vi "Teleop.vi"(10 "Match Info":T2={"Autonomous Elapsed Seconds"=0.0, "TeleOp Elapsed Seconds"=0.0, "Disabled Elapsed Seconds"=0.0, "Visited Autonomous"=FALSE, "Visited TeleOp"=FALSE, "Visited Disabled"=FALSE, "Autonomous Settings"={"Autonomous Style"=enum."Independent", "VI Refnum"=refnum}}, 11 "Call Context":T3) -> ()   [LabVIEW 2011]
doc: "This VI is called for each TeleOp packet received from the DS where the robot is not disabled. It is often used to read from the joysticks and update I/O or to update setpoints for timed control loops. It should complete and return within 20 milliseconds or it may miss DS packets."
uses:
  <vilib>/Rock Robotics/WPI/DriverStation/WPI_DriverStationDerivedRobotMode.ctl
  <vilib>/Rock Robotics/WPI/DriverStation/WPI_DriverStationMatch Info.ctl
  <vilib>/Rock Robotics/WPI/Relay/WPI_RelayValue.ctl
  Robot Global Data.vi
  <vilib>/ptbypt/NI_PtbyPt.lvlib
panel:
  in  "AutoSearch?":bool
  in  "MotorPower":dbl
  in  "Slide":dbl(slide) scale=400.0..2000.0
  out "Numeric":dbl
  out "Knob":dbl(knob) scale=0.0..360.0
  in  "RelayValue":T1
  out "Value 5":bool
  out "Value 4":bool
  out "Value 3":bool
  out "Value 2":bool
  out "Value":bool
  in  "top":bool=TRUE
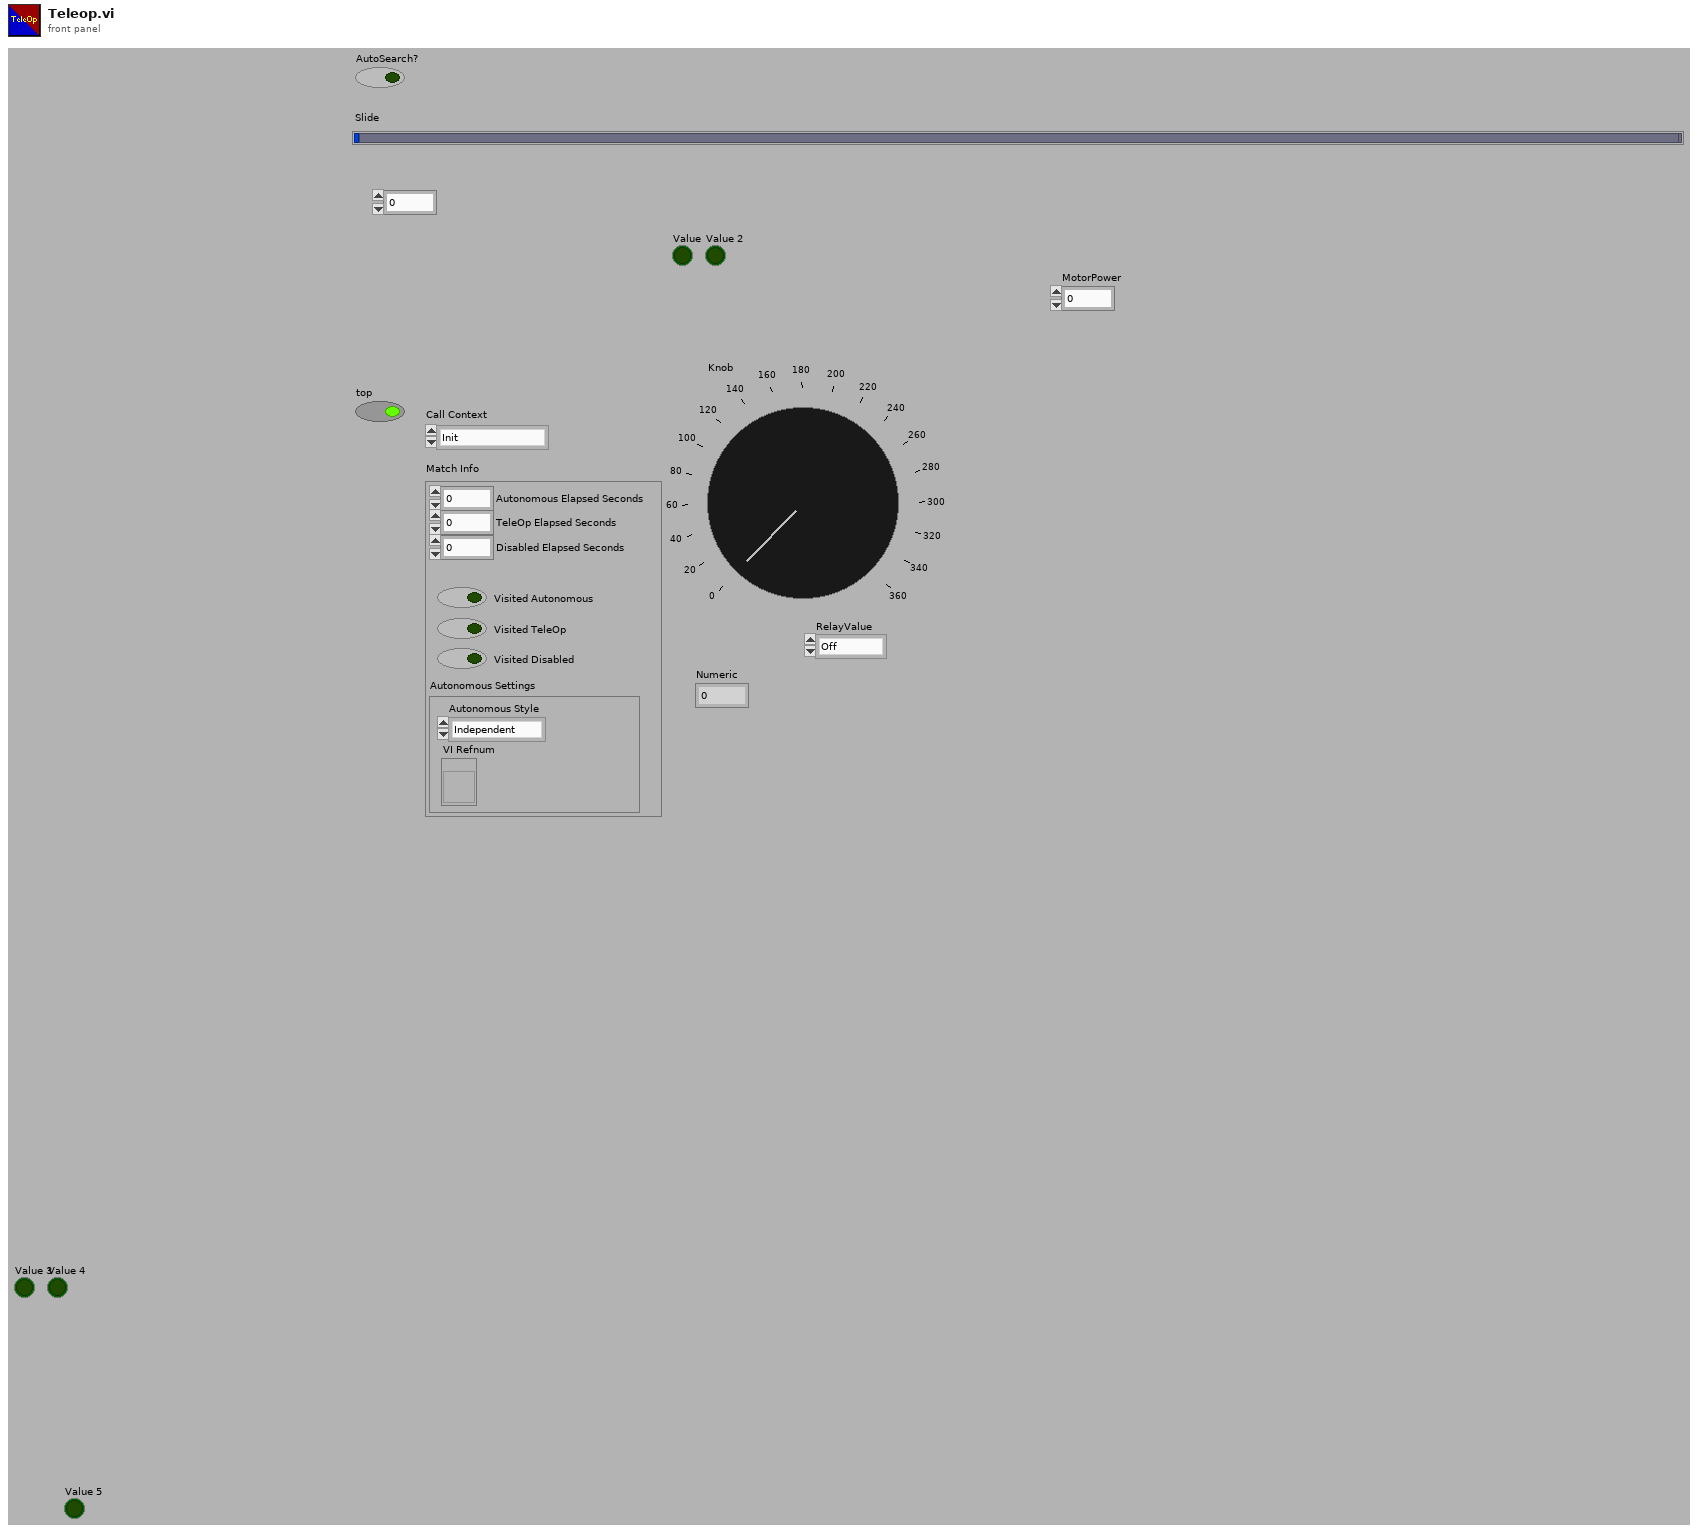
[diagram p1: front panel]
types:
  T1 = typedef "WPI_RelayValue.ctl" = enum16{"Off", "On", "Forward", "Reverse"}
  T2 = typedef "WPI_DriverStationMatch Info.ctl" = cluster{"Autonomous Elapsed Seconds":dbl, "TeleOp Elapsed Seconds":dbl, "Disabled Elapsed Seconds":dbl, "Visited Autonomous":bool, "Visited TeleOp":bool, "Visited Disabled":bool, "Autonomous Settings":cluster{"Autonomous Style":enum16{"Iterative", "Independent"}, "VI Refnum":refnum<vi>}}
  T3 = typedef "WPI_DriverStationDerivedRobotMode.ctl" = enum16{"Init", "Execute", "Stop"}
  T4 = typedef "WPI_RelayDevRef.ctl" = cluster{"DevStatus":errorcluster, "Relay Channel":T5, "Digital Module":T6, "Relay Direction":T7}
  T5 = typedef "FPGA_DIORelayChannel.ctl" = enum8{"Relay 1", "Relay 2", "Relay 3", "Relay 4", "Relay 5", "Relay 6", "Relay 7", "Relay 8", "Invalid"}
  T6 = typedef "FPGA_TypedefDigitalModule.ctl" = enum16{"Digital Module 1", "Digital Module 2"}
  T7 = typedef "WPI_RelayDirection.ctl" = enum16{"Both directions", "Forward only", "Reverse only"}
  T8 = typedef "WPI_AnalogChannelDevRef.ctl" = cluster{"DevStatus":errorcluster, "Analog Module":T9, "Analog Channel":T10}
  T9 = typedef "FPGA_TypedefAnalogModule.ctl" = enum16{"Analog Module 1", "Analog Module 2"}
  T10 = typedef "FPGA_AIChannel.ctl" = enum8{"AI 1", "AI 2", "AI 3", "AI 4", "AI 5", "AI 6", "AI 7", "AI 8", "Invalid"}
  T11 = typedef "WPI_DigitalInputDevRef.ctl" = cluster{"DevStatus":errorcluster, "DIO Channel":T12, "Digital Module":T6}
  T12 = typedef "FPGA_DIOChannel.ctl" = enum8{"DIO 1", "DIO 2", "DIO 3", "DIO 4", "DIO 5", "DIO 6", "DIO 7", "DIO 8", "DIO 9", "DIO 10", "DIO 11", "DIO 12", "DIO 13", "DIO 14", "Invalid"}
  T13 = cluster{"Position":cluster{"X":dbl, "Y":dbl}, "Distance (m)":dbl, "Target Found?":bool}
  T14 = typedef "WPI_ServoDeviceRef.ctl" = cluster{"DeviceStatus":errorcluster, "Digital Module":T6, "PWM Channel":T15, "DeadBand":T16}
  T15 = typedef "FPGA_DIOPWMChannel.ctl" = enum8{"PWM 1", "PWM 2", "PWM 3", "PWM 4", "PWM 5", "PWM 6", "PWM 7", "PWM 8", "PWM 9", "PWM 10", "Invalid"}
  T16 = typedef "WPI_PWMDeadband.ctl" = cluster{"Name":string, "maxPositivePwm":i32, "minPositivePwm":i32, "centerPwm":i32, "maxNegativePwm":i32, "minNegativePwm":i32, "angularRange":u16}
  T17 = typedef "WPI_MotorControlDeviceRef.ctl" = cluster{"DeviceStatus":errorcluster, "Type":enum16{"PWM", "CAN"}, "PWM":cluster{"Digital Module":T6, "PWM Channel":T15, "DeadBand":T16}, "CAN":cluster{"Device Number":u8, "Control Mode":T18, "Semaphore":T19, "Max Vout":dbl}, "Invert":bool, "TransformRef":T20, "InvTransformRef":T20}
  T18 = typedef "WPI_CANJaguar_ControlMode.ctl" = enum8{"Percent VBus", "Current", "Speed", "Position", "Voltage"}
  T19 = typedef "Semaphore RefNum" = refnum<k1>
  T20 = typedef "WPI_PWMTransform_ConPane.ctl" = refnum<vi>
  T21 = typedef "WPI_JoystickDevRef.ctl" = cluster{"Device":T22}
  T22 = typedef "WPI_JoystickDeviceEnum.ctl" = enum16{"USB 1", "USB 2", "USB 3", "USB 4", "Kinect 1", "Kinect 2"}
  T23 = typedef "WPI_EncoderDevRef.ctl" = cluster{"DevStatus":errorcluster, "EncoderIndex":T24, "CounterIndex":T25, "DistancePerCount":dbl, "Decoding Type":T26}
  T24 = typedef "FPGA_EncoderIdx.ctl" = enum8{"Enc 0", "Enc 1", "Enc 2", "Enc 3", "Invalid"}
  T25 = typedef "FPGA_CounterCtrSystemIndex.ctl" = enum8{"Ctr 0", "Ctr 1", "Ctr 2", "Ctr 3", "Ctr 4", "Ctr 5", "Ctr 6", "Ctr 7", "Invalid"}
  T26 = typedef "WPI_EncoderType.ctl" = enum16{"1x", "2x", "4x"}
  T27 = typedef "WPI_RobotDriveDevRef.ctl" = cluster{"DevStatus":errorcluster, "Motors[]":T17[], "Square Inputs":bool, "Max Output":dbl, "Isochronous":bool}
  T28 = typedef "WPI_GyroDevRef.ctl" = cluster{"DevStatus":errorcluster, "Analog Module":T9, "Analog Channel":T10, "Offset":dbl, "Gain (VoltsPerDegree/Second)":dbl}
  T29 = cluster{"axis 1 (x)":dbl, "axis 2 (y)":dbl, "axis 3 (throttle)":dbl, "axis 4":dbl, "axis 5":dbl, "axis 6":dbl}
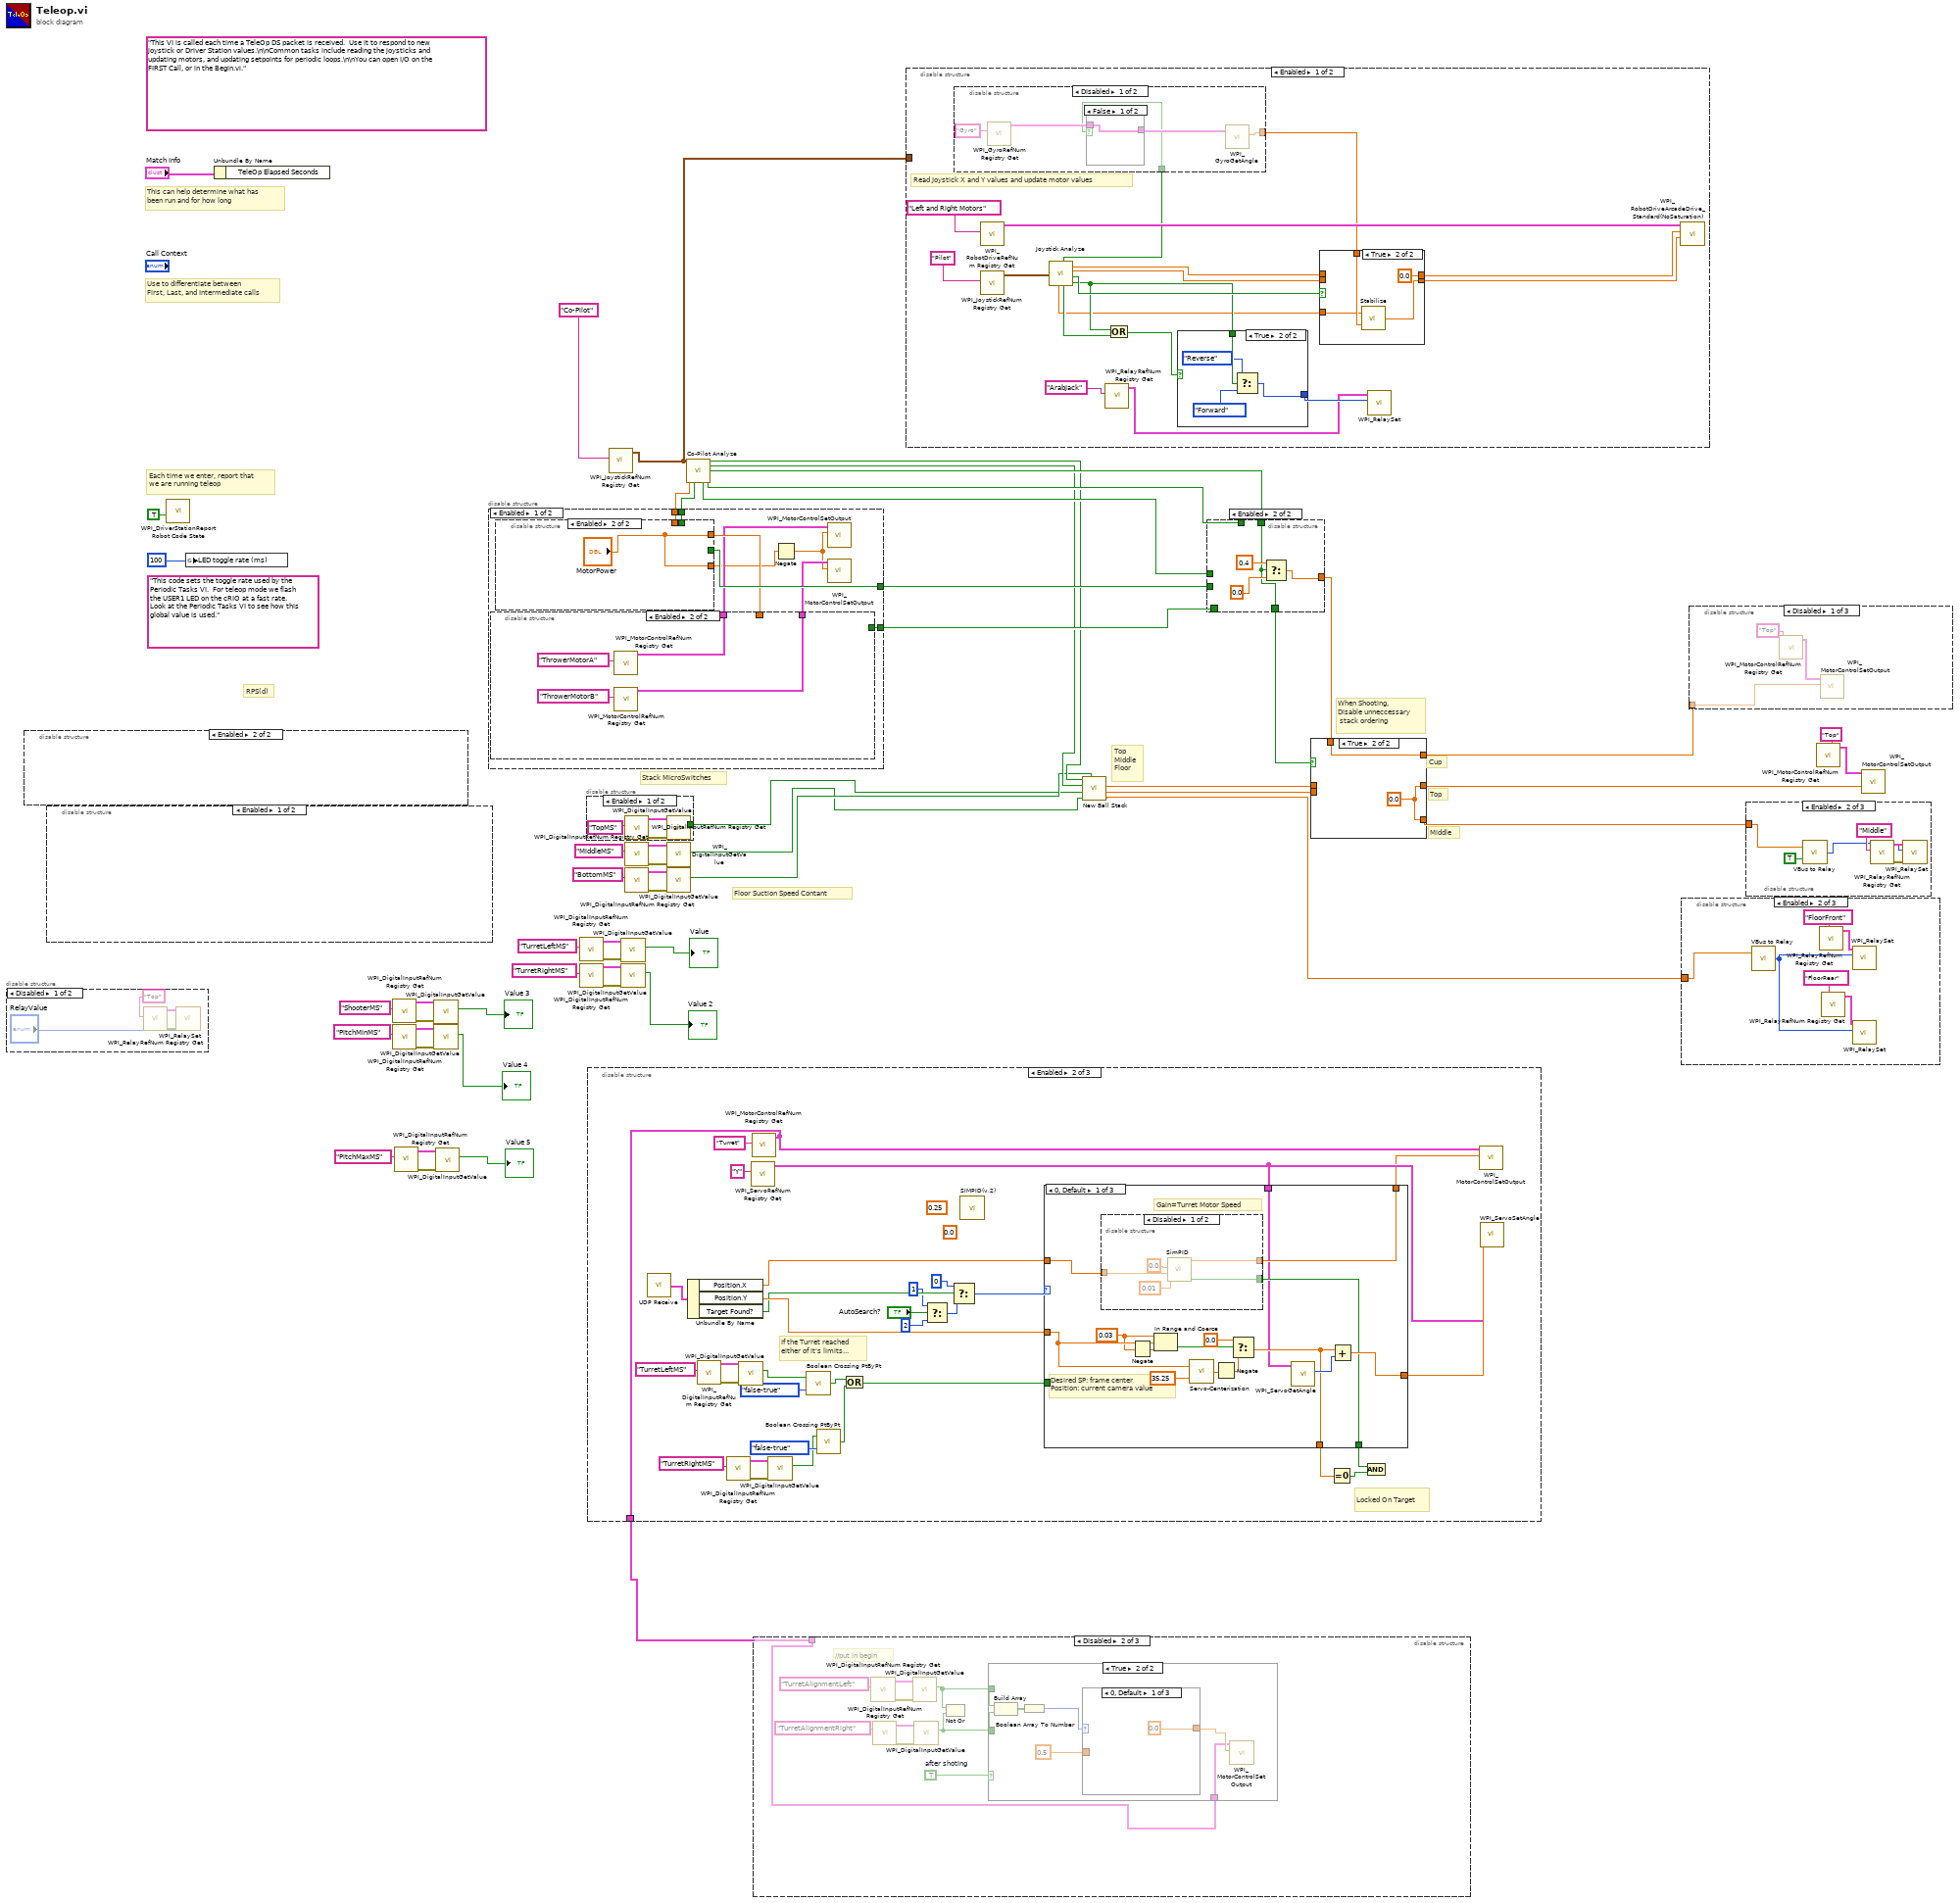
[diagram p0: block diagram]
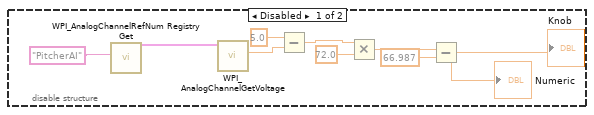
[diagram p2: hidden frame]
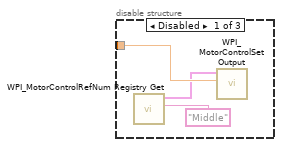
[diagram p5: hidden frame]
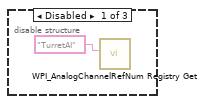
[diagram p7: hidden frame]
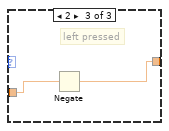
[diagram p10: hidden frame]
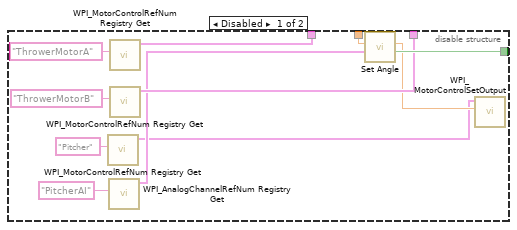
[diagram p12: hidden frame]
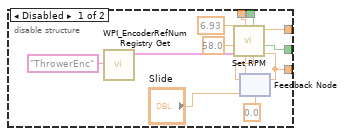
[diagram p13: hidden frame]
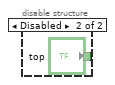
[diagram p15: hidden frame]
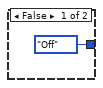
[diagram p16: hidden frame]
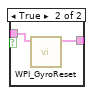
[diagram p17: hidden frame]
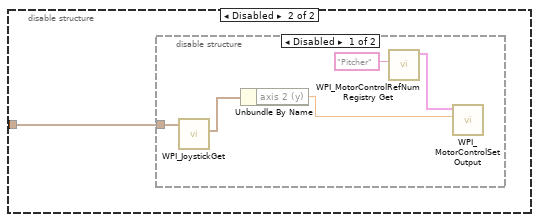
[diagram p20: hidden frame]
diagram:
  (unwired) "This code sets the toggle rate used by the Periodic Tasks VI.  For teleop mode we flash the USER1 LED on the cRIO at a fast rate.  Look at the Periodic Tasks VI to see how this global value is used."
  (unwired) "This VI is called each time a TeleOp DS packet is received.  Use it to respond to new joystick or Driver Station values.\n\nCommon tasks include reading the joysticks and updating motors, and updating setpoints for periodic loops.\n\nYou can open I/O on the FIRST Call, or in the Begin.vi."
  # "RPS(d)"
  # "Stack MicroSwitches"
  # "Top\nMiddle\nFloor"
  # "Floor Suction Speed Contant"
  # "When Shooting,\nDisable unneccessary\n stack ordering"
  # "Middle"
  # "Top"
  # "Cup"
  # "Each time we enter, report that\nwe are running teleop"
  # "Use to differentiate between\nFirst, Last, and Intermediate calls"
  # "This can help determine what has\nbeen run and for how long"
  n1 = disable-structure shown="Disabled" {
    frame Disabled {
      n2 = call <vilib>:"WPI_RelayRefNum Registry Get.vi"("refnum name"="Top") -> ("error out"=w56:errorcluster, "RelayDevRef"=w57:T4)  [unwired: 9 in]
      n3 = call <vilib>:"WPI_RelaySet.vi"("error in (no error)"=w56, "RelayValue"="RelayValue", "RelayDevRef"=w57) -> ()  [unwired: 7 in, 2 out]
    }
    frame Enabled {
    }
  }
  n4 = disable-structure shown="Enabled" {
    frame Disabled {
      n5 = call <vilib>:"WPI_AnalogChannelRefNum Registry Get.vi"("refnum name"="PitcherAI") -> ("AIDeviceRef"=w66:T8)  [unwired: 9 in, 1 out]
      n6 = call <vilib>:"WPI_AnalogChannelGetVoltage.vi"("AIDeviceRef"=w66) -> ("Voltage"=w60:dbl)  [unwired: 8 in, 2 out]
      n7 = Subtract(x=5.0, y=w60) -> (x-y=w59:dbl)
      n8 = Multiply(x=w59, y=72.0) -> (x*y=w64:dbl)
      n9 = Subtract(x=w64, y=66.987) -> (x-y=→"Knob" →"Numeric":dbl)
    }
    frame Enabled {
    }
  }
  n10 = disable-structure shown="Enabled" {
    frame Enabled {
    }
    frame Disabled {
    }
  }
  n11 = call <vilib>:"WPI_DriverStationReport Robot Code State.vi"("TeleOp"=TRUE ("Autonomous")) -> ()  [unwired: 10 in, 1 out]
  n12 = global write "Robot Global Data.vi" "LED toggle rate (ms)"(u32 100 ("LED ms toggle rate")) -> ()
  n13 = Unbundle By Name("Match Info") -> ()  [unwired: 1 out]
  n14 = call <vilib>:"WPI_DigitalInputRefNum Registry Get.vi"("refnum name"="ShooterMS") -> ("error out"=w20:errorcluster, "DigitalInputDevRef"=w17:T11)  [unwired: 9 in]
  n15 = call <vilib>:"WPI_DigitalInputRefNum Registry Get.vi"("refnum name"="PitchMinMS") -> ("error out"=w19:errorcluster, "DigitalInputDevRef"=w18:T11)  [unwired: 9 in]
  n16 = call <vilib>:"WPI_DigitalInputRefNum Registry Get.vi"("refnum name"="PitchMaxMS") -> ("error out"=w13:errorcluster, "DigitalInputDevRef"=w12:T11)  [unwired: 9 in]
  n17 = call <vilib>:"WPI_DigitalInputGetValue.vi"("error in (no error)"=w20, "DigitalInputDevRef"=w17) -> ("Value"=→"Value 3":bool)  [unwired: 7 in, 2 out]
  n18 = call <vilib>:"WPI_DigitalInputGetValue.vi"("error in (no error)"=w19, "DigitalInputDevRef"=w18) -> ("Value"=→"Value 4":bool)  [unwired: 7 in, 2 out]
  n19 = call <vilib>:"WPI_DigitalInputGetValue.vi"("error in (no error)"=w13, "DigitalInputDevRef"=w12) -> ("Value"=→"Value 5":bool)  [unwired: 7 in, 2 out]
  n20 = call <vilib>:"WPI_DigitalInputRefNum Registry Get.vi"("refnum name"="TurretLeftMS") -> ("error out"=w28:errorcluster, "DigitalInputDevRef"=w25:T11)  [unwired: 9 in]
  n21 = call <vilib>:"WPI_DigitalInputRefNum Registry Get.vi"("refnum name"="TurretRightMS") -> ("error out"=w27:errorcluster, "DigitalInputDevRef"=w26:T11)  [unwired: 9 in]
  n22 = disable-structure shown="Enabled" {
    disable-tunnel: [w68 "top"] -> w5
    frame Enabled {
      n23 = call <vilib>:"WPI_DigitalInputRefNum Registry Get.vi"("refnum name"="TopMS") -> ("error out"=w70:errorcluster, "DigitalInputDevRef"=w69:T11)  [unwired: 9 in]
      n24 = call <vilib>:"WPI_DigitalInputGetValue.vi"("error in (no error)"=w70, "DigitalInputDevRef"=w69) -> ("Value"=w68:bool)  [unwired: 7 in, 2 out]
    }
    frame Disabled {
    }
  }
  n25 = disable-structure shown="Enabled" {
    disable-tunnel: [_ w140 _] -> w33
    frame Disabled {
      # "Locked On Target"
      # "Enable Auto Search"
      n26 = call "UDP Receive.vi"() -> ("Selected Target Info"=w88:T13)  [unwired: 1 in]
      n27 = Unbundle By Name(w88) -> ("Position.X"=w84:dbl, "Position.Y"=w83:dbl, "Target Found?"=w74:bool)  [unwired: 1 out]
      n28 = call <vilib>:"WPI_ServoRefNum Registry Get.vi"("refnum name"="Y") -> ("ServoDeviceRef"=w81:T14)  [unwired: 9 in, 1 out]
      n29 = call <vilib>:"WPI_ServoRefNum Registry Get.vi"("refnum name"="X") -> ("ServoDeviceRef"=w82:T14)  [unwired: 9 in, 1 out]
      n30 = Not(x=w74) -> (.not. x?=w73:bool)
      n31 = Compound Arithmetic op=AND(w73, TRUE ("y")) -> (w75:bool)
      n32 = case shown="False" w75 {
        tunnel: [w94 w119] -> w80
        tunnel: [w93 w113] -> w85
        tunnel: w83 -> [w102 _]
        tunnel: w84 -> [w99 _]
        tunnel: w82 -> [w92 _]
        tunnel: w81 -> [w91 _]
        tunnel: [w90 w112] -> w79
        tunnel: [w89 w112] -> w78
        frame False {
          w98 = 0.01 ("lower limit")
          w100 = 0.01 ("upper limit")
          n33 = Negate(x=w100) -> (-x=w101:dbl)
          n34 = Negate(x=w98) -> (-x=w97:dbl)
          n35 = In Range and Coerce(upper limit=w100, x=w99, lower limit=w101) -> (In Range?=w103:bool)  [unwired: 1 out]
          n36 = In Range and Coerce(upper limit=w98, x=w102, lower limit=w97) -> (In Range?=w104:bool)  [unwired: 1 out]
          n37 = call "Servo-Centerization.vi"("Camera Angle"=47.0 ("HALF Cam angle constant"), "Cartez"=w99) -> ("Rounded Error"=w106:dbl)
          n38 = call "Servo-Centerization.vi"("Camera Angle"=35.25 ("HALF Cam angle constant"), "Cartez"=w102) -> ("Rounded Error"=w110:dbl)
          n39 = Negate(x=w110) -> (-x=w111:dbl)
          n40 = Select(t=0.0 ("f"), s=w103, f=w106) -> (s? t:f=w90:dbl)
          n41 = Select(t=0.0 ("f"), s=w104, f=w111) -> (s? t:f=w89:dbl)
          n42 = call <vilib>:"WPI_ServoGetAngle.vi"("ServoDeviceRef"=w91) -> ("Angle"=w96:u16)  [unwired: 7 in, 2 out]
          n43 = call <vilib>:"WPI_ServoGetAngle.vi"("ServoDeviceRef"=w92) -> ("Angle"=w95:u16)  [unwired: 7 in, 2 out]
          n44 = Add(x=w89, y=w96) -> (x+y=w93:dbl)
          n45 = Add(x=w90, y=w95) -> (x+y=w94:dbl)
        }
        frame True {
          w112 = 1.0 ("Rounded Error")
          n46 = feedback #1(0.0 ("counter")) -> (w117:dbl)
          n47 = call "Auto-Search.vi"("Counter\\Timer"=w117, "Low Angle Edge"=30.0, "High Angle Edge"=130.0) -> ("counter"=w116:dbl, "Servo Angle"=w113:dbl)
          n48 = feedback-in #1(w116) -> ()
          n49 = feedback #2(0.0 ("counter")) -> (w121:dbl)
          n50 = call "Auto-Search.vi"("Counter\\Timer"=w121, "Low Angle Edge"=30.0, "High Angle Edge"=130.0) -> ("counter"=w122:dbl, "Servo Angle"=w119:dbl)
          n51 = feedback-in #2(w122) -> ()
        }
      }
      n52 = Add(x=w79, y=w78) -> (x+y=w77:dbl)
      n53 = Equal To 0?(x=w77) -> ()  [unwired: 1 out]
      n54 = call <vilib>:"WPI_ServoSetAngle.vi"("Angle"=w80, "ServoDeviceRef"=w82) -> ()  [unwired: 8 in, 2 out]
      n55 = call <vilib>:"WPI_ServoSetAngle.vi"("Angle"=w85, "ServoDeviceRef"=w81) -> ()  [unwired: 8 in, 2 out]
    }
    frame Enabled {
      (unwired) 0.0 ("Set Point")
      (unwired) 0.25 ("Gain")
      # "If the Turret reached \neither of it's limits..."
      # "Locked On Target"
      n56 = call "UDP Receive.vi"() -> ("Selected Target Info"=w156:T13)  [unwired: 1 in]
      n57 = Unbundle By Name(w156) -> ("Position.X"=w131:dbl, "Position.Y"=w153:dbl, "Target Found?"=w130:bool)
      n58 = call <vilib>:"WPI_DigitalInputRefNum Registry Get.vi"("refnum name"="TurretLeftMS") -> ("error out"=w145:errorcluster, "DigitalInputDevRef"=w141:T11)  [unwired: 9 in]
      n59 = call <vilib>:"WPI_DigitalInputRefNum Registry Get.vi"("refnum name"="TurretRightMS") -> ("error out"=w144:errorcluster, "DigitalInputDevRef"=w143:T11)  [unwired: 9 in]
      n60 = call <vilib>:"WPI_DigitalInputGetValue.vi"("error in (no error)"=w145, "DigitalInputDevRef"=w141) -> ("Value"=w137:bool)  [unwired: 7 in, 2 out]
      n61 = call <vilib>:"WPI_ServoRefNum Registry Get.vi"("refnum name"="Y") -> ("ServoDeviceRef"=w152:T14)  [unwired: 9 in, 1 out]
      n62 = call <vilib>:"WPI_MotorControlRefNum Registry Get.vi"("refnum name"="Turret") -> ("MotorControlDevRef"=w140:T17)  [unwired: 9 in, 1 out]
      n63 = call <vilib>:"WPI_DigitalInputGetValue.vi"("error in (no error)"=w144, "DigitalInputDevRef"=w143) -> ("Value"=w134:bool)  [unwired: 7 in, 2 out]
      n64 = call <vilib>:"Boolean Crossing PtByPt.vi"("direction"=enum16{"either", "false-true", "true-false"}."false-true", "input"=w137) -> ("crossing"=w136:bool)  [unwired: 1 in]
      n65 = call <vilib>:"Boolean Crossing PtByPt.vi"("direction"=enum16{"either", "false-true", "true-false"}."false-true", "input"=w134) -> ("crossing"=w133:bool)  [unwired: 1 in]
      n66 = Or(x=w136, y=w133) -> (x .or. y?=w142:bool)
      n67 = Select(t=1 ("Position.X"), s="AutoSearch?", f=2 ("Position.X")) -> (s? t:f=w132:i32)
      n68 = Select(t=0 ("Position.X"), s=w130, f=w132) -> (s? t:f=w125:i32)
      n69 = call "SIMPID(v.2).vi"() -> ()  [unwired: 10 in, 2 out]
      n70 = case shown="0, Default" w125 {
        tunnel: [w162 w181 0.0 ("Servo Angle")] -> w154
        tunnel: w153 -> [w166 _ _]
        tunnel: w131 -> [w160 _ _]
        tunnel: w152 -> [w157 _ _]
        tunnel: [w161 1.0 ("Rounded Error") 1.0 ("Rounded Error")] -> w150
        tunnel: [w159 FALSE ("On Target") FALSE ("On Target")] -> w148
        tunnel: [w158 w177 0.0 ("t")] -> w139
        tunnel: w142 -> [_ w178 _]
        frame 0, Default {
          w165 = 0.03 ("lower limit")
          # "Desired SP: frame center\nPosition: current camera value"
          # "Gain=Turret Motor Speed"
          n71 = disable-structure shown="Disabled" {
            disable-tunnel: w160 -> [w176 _]
            disable-tunnel: [w173 _] -> w159
            disable-tunnel: [w172 _] -> w158
            frame Disabled {
              n72 = call "SimPID.vi"("Range"=0.01, "Position"=w176, "Set Point"=0.0) -> ("On Target"=w173:bool, "result"=w172:dbl)  [unwired: 6 in]
            }
            frame Enabled {
            }
          }
          n73 = Negate(x=w165) -> (-x=w164:dbl)
          n74 = In Range and Coerce(upper limit=w165, x=w166, lower limit=w164) -> (In Range?=w167:bool)  [unwired: 1 out]
          n75 = call "Servo-Centerization.vi"("Camera Angle"=35.25 ("HALF Cam angle constant"), "Cartez"=w166) -> ("Rounded Error"=w170:dbl)
          n76 = Negate(x=w170) -> (-x=w171:dbl)
          n77 = Select(t=0.0 ("f"), s=w167, f=w171) -> (s? t:f=w161:dbl)
          n78 = call <vilib>:"WPI_ServoGetAngle.vi"("ServoDeviceRef"=w157) -> ("Angle"=w163:u16)  [unwired: 7 in, 2 out]
          n79 = Add(x=w161, y=w163) -> (x+y=w162:dbl)
        }
        frame 1 {
          n80 = disable-structure shown="Disabled" {
            disable-tunnel: w178 -> [w191 _]
            disable-tunnel: [w187 _] -> w177
            frame Disabled {
              w189 = -0.11 ("t")
              # "If either of the MS's are pressed,\nthe latched boolean value will affect\nthe value Select returns so that\nit'd go in the other direction."
              # "Turret Motor Speed"
              n81 = call "Button2Toggle.vi"("Boolean"=w191) -> ("Latched Boolean"=w190:bool)  [unwired: 9 in, 1 out]
              n82 = Negate(x=w189) -> (-x=w188:dbl)
              n83 = Select(t=w189, s=w190, f=w188) -> (s? t:f=w187:dbl)
            }
            frame Enabled {
            }
          }
          n84 = feedback #3(0.0 ("counter")) -> (w185:dbl)
          n85 = call "Auto-Search.vi"("Counter\\Timer"=w185, "Low Angle Edge"=90.0, "High Angle Edge"=110.0) -> ("counter"=w184:dbl, "Servo Angle"=w181:dbl)
          n86 = feedback-in #3(w184) -> ()
        }
        frame 2 {
        }
      }
      n87 = Equal To 0?(x=w150) -> (x = 0?=w149:bool)
      n88 = And(x=w148, y=w149) -> ()  [unwired: 1 out]
      n89 = call <vilib>:"WPI_MotorControlSetOutput.vi"("Output"=w139, "MotorControlDevRef"=w140) -> ()  [unwired: 8 in, 2 out]
      n90 = call <vilib>:"WPI_ServoSetAngle.vi"("Angle"=w154, "ServoDeviceRef"=w152) -> ()  [unwired: 8 in, 2 out]
    }
    frame Disabled {
    }
  }
  n91 = call <vilib>:"WPI_JoystickRefNum Registry Get.vi"("refnum name"="Co-Pilot") -> ("JoystickDevRef"=w9:T21)  [unwired: 1 in, 9 out]
  n92 = call <vilib>:"WPI_DigitalInputGetValue.vi"("error in (no error)"=w28, "DigitalInputDevRef"=w25) -> ("Value"=→"Value":bool)  [unwired: 7 in, 2 out]
  n93 = call <vilib>:"WPI_DigitalInputGetValue.vi"("error in (no error)"=w27, "DigitalInputDevRef"=w26) -> ("Value"=→"Value 2":bool)  [unwired: 7 in, 2 out]
  n94 = call <vilib>:"WPI_DigitalInputRefNum Registry Get.vi"("refnum name"="MiddleMS") -> ("error out"=w43:errorcluster, "DigitalInputDevRef"=w42:T11)  [unwired: 9 in]
  n95 = call <vilib>:"WPI_DigitalInputRefNum Registry Get.vi"("refnum name"="BottomMS") -> ("error out"=w41:errorcluster, "DigitalInputDevRef"=w40:T11)  [unwired: 9 in]
  n96 = call <vilib>:"WPI_DigitalInputGetValue.vi"("error in (no error)"=w43, "DigitalInputDevRef"=w42) -> ("Value"=w4:bool)  [unwired: 7 in, 2 out]
  n97 = call <vilib>:"WPI_DigitalInputGetValue.vi"("error in (no error)"=w41, "DigitalInputDevRef"=w40) -> ("Value"=w6:bool)  [unwired: 7 in, 2 out]
  n98 = call "Co-Pilot Analyze.vi"("JoystickDevRef"=w9) -> ("Suction"=w8:bool, "Ejection"=w7:bool, "Button 6"=w10:bool, "Fine Tune(RPM)"=w36:dbl, "Fine Tune?"=w35:bool, "Fire Override"=w37:bool, "Fire"=w38:bool)  [unwired: 8 in]
  n99 = disable-structure shown="Enabled" {
    disable-tunnel: [w204 _] -> w51
    disable-tunnel: w36 -> [w203 _]
    disable-tunnel: w35 -> [w202 _]
    disable-tunnel: [w201 _] -> w34
    frame Enabled {
      n100 = disable-structure shown="Enabled" {
        disable-tunnel: [w231 _] -> w204
        disable-tunnel: w203 -> [w228 _]
        disable-tunnel: w202 -> [w227 _]
        disable-tunnel: [w224 "MotorPower"] -> w200
        disable-tunnel: [w223 "MotorPower"] -> w197
        frame Disabled {
          n101 = call <vilib>:"WPI_EncoderRefNum Registry Get.vi"("refnum name"="ThrowerEnc") -> ("EncoderDevRef"=w230:T23)  [unwired: 9 in, 1 out]
          n102 = feedback #4(0.0 ("Thrower Voltage")) -> (w226:dbl)
          n103 = call "Set RPM.vi"("Last Thrower Voltage (node)"=w226, "Fine Tune?"=w227, "Position"="Slide", "Fine Tuning"=w228, "EncoderDevRef"=w230, "Angle"=58.0, "horizontal distance to basket"=6.93) -> ("Thrower Voltage"=w223:dbl, "RPM SET"=w231:bool, "angle"=w224:dbl)  [unwired: 2 in]
          n104 = feedback-in #4(w223) -> ()
        }
        frame Enabled {
        }
      }
      n105 = disable-structure shown="Enabled" {
        disable-tunnel: [w215 _] -> w201
        disable-tunnel: w200 -> [w214 _]
        disable-tunnel: [w211 w217] -> w199
        disable-tunnel: [w210 w216] -> w198
        frame Disabled {
          n106 = call <vilib>:"WPI_MotorControlRefNum Registry Get.vi"("refnum name"="Pitcher") -> ("MotorControlDevRef"=w205:T17)  [unwired: 9 in, 1 out]
          n107 = call <vilib>:"WPI_AnalogChannelRefNum Registry Get.vi"("refnum name"="PitcherAI") -> ("AIDeviceRef"=w207:T8)  [unwired: 9 in, 1 out]
          n108 = call <vilib>:"WPI_MotorControlRefNum Registry Get.vi"("refnum name"="ThrowerMotorA") -> ("MotorControlDevRef"=w211:T17)  [unwired: 9 in, 1 out]
          n109 = call <vilib>:"WPI_MotorControlRefNum Registry Get.vi"("refnum name"="ThrowerMotorB") -> ("MotorControlDevRef"=w210:T17)  [unwired: 9 in, 1 out]
          n110 = call "Set Angle.vi"("AIDeviceRef"=w207, "Angle"=w214) -> ("Angle SET"=w215:bool, "Angle Motor"=w206:dbl)  [unwired: 8 in]
          n111 = call <vilib>:"WPI_MotorControlSetOutput.vi"("Output"=w206, "MotorControlDevRef"=w205) -> ()  [unwired: 8 in, 2 out]
        }
        frame Enabled {
          n112 = call <vilib>:"WPI_MotorControlRefNum Registry Get.vi"("refnum name"="ThrowerMotorA") -> ("MotorControlDevRef"=w217:T17)  [unwired: 9 in, 1 out]
          n113 = call <vilib>:"WPI_MotorControlRefNum Registry Get.vi"("refnum name"="ThrowerMotorB") -> ("MotorControlDevRef"=w216:T17)  [unwired: 9 in, 1 out]
        }
      }
      n114 = Negate(x=w197) -> (-x=w196:dbl)
      n115 = call <vilib>:"WPI_MotorControlSetOutput.vi"("Output"=w196, "MotorControlDevRef"=w199) -> ()  [unwired: 8 in, 2 out]
      n116 = call <vilib>:"WPI_MotorControlSetOutput.vi"("Output"=w196, "MotorControlDevRef"=w198) -> ()  [unwired: 8 in, 2 out]
    }
    frame Disabled {
    }
  }
  n117 = disable-structure shown="Disabled" {
    disable-tunnel: w33 -> [_ w234 _]
    frame Disabled {
      n118 = call <vilib>:"WPI_AnalogChannelRefNum Registry Get.vi"("refnum name"="TurretAI") -> ()  [unwired: 9 in, 2 out]
    }
    frame Disabled {
      w235 = TRUE  # after shoting
      # "//put in begin"
      n119 = call <vilib>:"WPI_DigitalInputRefNum Registry Get.vi"("refnum name"="TurretAlignmentLeft") -> ("error out"=w242:errorcluster, "DigitalInputDevRef"=w241:T11)  [unwired: 9 in]
      n120 = call <vilib>:"WPI_DigitalInputRefNum Registry Get.vi"("refnum name"="TurretAlignmentRight") -> ("error out"=w239:errorcluster, "DigitalInputDevRef"=w240:T11)  [unwired: 9 in]
      n121 = call <vilib>:"WPI_DigitalInputGetValue.vi"("error in (no error)"=w242, "DigitalInputDevRef"=w241) -> ("Value"=w237:bool)  [unwired: 7 in, 2 out]
      n122 = call <vilib>:"WPI_DigitalInputGetValue.vi"("error in (no error)"=w239, "DigitalInputDevRef"=w240) -> ("Value"=w236:bool)  [unwired: 7 in, 2 out]
      n123 = Not Or(1:w236, 2:w237) -> ()  [unwired: 1 out]
      n124 = case shown="True" w235 {
        tunnel: w237 -> [_ w250]
        tunnel: w236 -> [_ w249]
        tunnel: w234 -> [_ w244]
        frame False {
        }
        frame True {
          n125 = Build Array(w250, w249) -> (w248:bool[])
          n126 = Boolean Array To Number(Boolean array=w248) -> (number=w247:u32)
          n127 = case shown="0, Default" w247 {
            tunnel: [0.0 w252 w253] -> w245
            tunnel: 0.5 -> [_ w252 w254]
            frame 0, Default {
            }
            frame 1 {
              # "right pressed"
            }
            frame 2 {
              # "left pressed"
              n128 = Negate(x=w254) -> (-x=w253:dbl)
            }
          }
          n129 = call <vilib>:"WPI_MotorControlSetOutput.vi"("Output"=w245, "MotorControlDevRef"=w244) -> ()  [unwired: 8 in, 2 out]
        }
      }
    }
    frame Enabled {
    }
  }
  n130 = disable-structure shown="Enabled" {
    disable-tunnel: w9 -> [_ w292]
    frame Enabled {
      # "Read Joystick X and Y values and update motor values"
      n131 = call <vilib>:"WPI_RobotDriveRefNum Registry Get.vi"("refnum name"="Left and Right Motors") -> ("RobotDriveDevRef"=w271:T27)  [unwired: 1 in, 9 out]
      n132 = call <vilib>:"WPI_JoystickRefNum Registry Get.vi"("refnum name"="Pilot") -> ("JoystickDevRef"=w269:T21)  [unwired: 1 in, 9 out]
      n133 = call "Joystick Analyze.vi"("Joystick Name"=w269) -> ("Stabilize Gain"=w255:dbl, "ResetGyro"=w256:bool, "x"=w266:dbl, "y"=w267:dbl, "Open Jack"=w261:bool, "Stabilize"=w264:bool, "Close Jack"=w260:bool)  [unwired: 3 in]
      n134 = disable-structure shown="Disabled" {
        disable-tunnel: [w281 _] -> w263
        disable-tunnel: w256 -> [w278 _]
        frame Disabled {
          n135 = call <vilib>:"WPI_GyroRefNum Registry Get.vi"("refnum name"="Gyro") -> ("GyroDevRef"=w280:T28)  [unwired: 9 in, 1 out]
          n136 = case shown="False" w278 {
            tunnel: w280 -> [w283 w285]
            tunnel: [w283 w284] -> w279
            frame False {
            }
            frame True {
              n137 = call <vilib>:"WPI_GyroReset.vi"("GyroDevRef"=w285) -> ("GyroDevRef"=w284:T28)  [unwired: 9 in, 1 out]
            }
          }
          n138 = call <vilib>:"WPI_GyroGetAngle.vi"("GyroDevRef"=w279) -> ("Angle"=w281:dbl)  [unwired: 7 in, 3 out]
        }
        frame Enabled {
        }
      }
      n139 = call <vilib>:"WPI_RelayRefNum Registry Get.vi"("refnum name"="ArabJack") -> ("RelayDevRef"=w258:T4)  [unwired: 9 in, 1 out]
      n140 = Or(x=w260, y=w261) -> (x .or. y?=w257:bool)
      n141 = case shown="True" w257 {
        tunnel: w260 -> [_ w277]
        tunnel: [WPI_RelayValue."Off" ("RelayValue") w274] -> w259
        frame False {
        }
        frame True {
          n142 = Select(t=WPI_RelayValue."Reverse" ("RelayValue"), s=w277, f=WPI_RelayValue."Forward" ("RelayValue")) -> (s? t:f=w274:T1)
        }
      }
      n143 = case shown="True" w264 {
        tunnel: [w287 w290] -> w268
        tunnel: w267 -> [w287 _]
        tunnel: [w286 0.0 ("x")] -> w265
        tunnel: w266 -> [w286 _]
        tunnel: w263 -> [_ w289]
        tunnel: w255 -> [_ w288]
        frame False {
        }
        frame True {
          n144 = call "Stabilize.vi"("Angle"=w289, "Gain"=w288) -> ("result"=w290:dbl)
        }
      }
      n145 = call <vilib>:"WPI_RelaySet.vi"("RelayValue"=w259, "RelayDevRef"=w258) -> ()  [unwired: 8 in, 2 out]
      n146 = call <vilib>:"WPI_RobotDriveArcadeDrive_Standard(NoSaturation).vi"("Y axis value"=w268, "X axis value"=w265, "RobotDriveDevRef"=w271) -> ()  [unwired: 1 in, 8 out]
    }
    frame Disabled {
      n147 = disable-structure shown="Disabled" {
        disable-tunnel: w292 -> [w296 _]
        frame Disabled {
          n148 = call <vilib>:"WPI_JoystickGet.vi"("JoystickDevRef"=w296) -> ("Axes"=w297:T29)  [unwired: 4 in, 2 out]
          n149 = Unbundle By Name(w297) -> ("axis 2 (y)"=w295:dbl)
          n150 = call <vilib>:"WPI_MotorControlRefNum Registry Get.vi"("refnum name"="Pitcher") -> ("MotorControlDevRef"=w294:T17)  [unwired: 9 in, 1 out]
          n151 = call <vilib>:"WPI_MotorControlSetOutput.vi"("Output"=w295, "MotorControlDevRef"=w294) -> ()  [unwired: 8 in, 2 out]
        }
        frame Enabled {
        }
      }
    }
  }
  n152 = call "New Ball Stack.vi"("BottomMS"=w6, "TopMS"=w4, "CupMS"=w5, "spinOut?"=w7, "Suck?"=w8) -> ("Floor"=w3:dbl, "Middle"=w2:dbl, "Top"=w1:dbl)  [unwired: 2 in]
  n153 = disable-structure shown="Enabled" {
    disable-tunnel: w51 -> [w300 _]
    disable-tunnel: [w304 w305] -> w50
    disable-tunnel: [w303 w306] -> w49
    disable-tunnel: w38 -> [w302 _]
    disable-tunnel: w37 -> [w301 _]
    disable-tunnel: w34 -> [w298 _]
    disable-tunnel: w10 -> [_ w305]
    frame Disabled {
      n154 = Compound Arithmetic op=AND(w300, w298) -> (w299:bool)  [unwired: 1 in]
      n155 = call "Shoot.vi"("Ready 2 Shoot?"=w299, "Fire"=w302, "Override"=w301) -> ("Le Fire at Will?"=w304:bool, "Top"=w303:dbl)  [unwired: 1 in]
    }
    frame Enabled {
      n156 = Select(t=0.4, s=w305, f=0.0 ("t")) -> (s? t:f=w306:dbl)
    }
  }
  n157 = case shown="True" w50 {
    tunnel: [0.0 ("Top") w313] -> w48
    tunnel: w49 -> [_ w313]
    tunnel: [w311 w312] -> w32
    tunnel: [w310 w312] -> w31
    tunnel: w2 -> [w310 _]
    tunnel: w1 -> [w311 _]
    frame False {
    }
    frame True {
      w312 = 0.0 ("Top")
    }
  }
  n158 = disable-structure shown="Enabled" {
    disable-tunnel: w3 -> [w314 w318 _]
    frame Disabled {
      n159 = call <vilib>:"WPI_MotorControlRefNum Registry Get.vi"("refnum name"="Floor") -> ("MotorControlDevRef"=w315:T17)  [unwired: 9 in, 1 out]
      n160 = call <vilib>:"WPI_MotorControlSetOutput.vi"("Output"=w314, "MotorControlDevRef"=w315) -> ()  [unwired: 8 in, 2 out]
    }
    frame Enabled {
      n161 = call "VBus to Relay.vi"("Motor VBus"=w318) -> ("RelayValue"=w317:T1)  [unwired: 1 in]
      n162 = call <vilib>:"WPI_RelayRefNum Registry Get.vi"("refnum name"="FloorFront") -> ("RelayDevRef"=w322:T4)  [unwired: 9 in, 1 out]
      n163 = call <vilib>:"WPI_RelayRefNum Registry Get.vi"("refnum name"="FloorRear") -> ("RelayDevRef"=w319:T4)  [unwired: 9 in, 1 out]
      n164 = call <vilib>:"WPI_RelaySet.vi"("RelayValue"=w317, "RelayDevRef"=w322) -> ()  [unwired: 8 in, 2 out]
      n165 = call <vilib>:"WPI_RelaySet.vi"("RelayValue"=w317, "RelayDevRef"=w319) -> ()  [unwired: 8 in, 2 out]
    }
    frame Disabled {
    }
  }
  n166 = disable-structure shown="Disabled" {
    disable-tunnel: w48 -> [w325 w326 _]
    frame Disabled {
      n167 = call <vilib>:"WPI_MotorControlRefNum Registry Get.vi"("refnum name"="Top") -> ("MotorControlDevRef"=w324:T17)  [unwired: 9 in, 1 out]
      n168 = call <vilib>:"WPI_MotorControlSetOutput.vi"("Output"=w325, "MotorControlDevRef"=w324) -> ()  [unwired: 8 in, 2 out]
    }
    frame Enabled {
      n169 = call "VBus to Relay.vi"("Motor VBus"=w326) -> ("RelayValue"=w327:T1)  [unwired: 1 in]
      n170 = call <vilib>:"WPI_RelayRefNum Registry Get.vi"("refnum name"="Cup") -> ("error out"=w328:errorcluster, "RelayDevRef"=w329:T4)  [unwired: 9 in]
      n171 = call <vilib>:"WPI_RelaySet.vi"("error in (no error)"=w328, "RelayValue"=w327, "RelayDevRef"=w329) -> ()  [unwired: 7 in, 2 out]
    }
    frame Disabled {
    }
  }
  n172 = disable-structure shown="Enabled" {
    disable-tunnel: w31 -> [w333 w336 _]
    frame Disabled {
      n173 = call <vilib>:"WPI_MotorControlRefNum Registry Get.vi"("refnum name"="Middle") -> ("MotorControlDevRef"=w331:T17)  [unwired: 9 in, 1 out]
      n174 = call <vilib>:"WPI_MotorControlSetOutput.vi"("Output"=w333, "MotorControlDevRef"=w331) -> ()  [unwired: 8 in, 2 out]
    }
    frame Enabled {
      n175 = call "VBus to Relay.vi"("Invert Relay? (F)"=TRUE, "Motor VBus"=w336) -> ("RelayValue"=w334:T1)
      n176 = call <vilib>:"WPI_RelayRefNum Registry Get.vi"("refnum name"="Middle") -> ("error out"=w337:errorcluster, "RelayDevRef"=w338:T4)  [unwired: 9 in]
      n177 = call <vilib>:"WPI_RelaySet.vi"("error in (no error)"=w337, "RelayValue"=w334, "RelayDevRef"=w338) -> ()  [unwired: 7 in, 2 out]
    }
    frame Disabled {
    }
  }
  n178 = call <vilib>:"WPI_MotorControlRefNum Registry Get.vi"("refnum name"="Top") -> ("MotorControlDevRef"=w47:T17)  [unwired: 9 in, 1 out]
  n179 = call <vilib>:"WPI_MotorControlSetOutput.vi"("Output"=w32, "MotorControlDevRef"=w47) -> ()  [unwired: 8 in, 2 out]
